vi "Write_INI.vi"(8 "error in (no error)":errorcluster, 10 "Options":T1={"Form_data_log_period"=0, "startup_threshold"=0.0, "Coeff_U"=2.55, "Offset_U"=6.5, "Coeff_I"=42.391, "Offset_I"=77.0, "Save_data_path"=path "", "ADC_frequency"=50000.0, "VISA resource name"="COM1"}, 11 "Ini_file_path":path) -> (0 "error out":errorcluster, 3 "Ini_file_path_out":path)   [LabVIEW 2012]
uses:
  Controls/options.ctl
  <vilib>/Utility/config.llb/Write Key (I32).vi
  <vilib>/Utility/config.llb/Write Key (Double).vi
  <vilib>/Utility/config.llb/Write Key (Path).vi
  <vilib>/Utility/config.llb/Write Key (String).vi
  <vilib>/Utility/config.llb/NI_LVConfig.lvlib
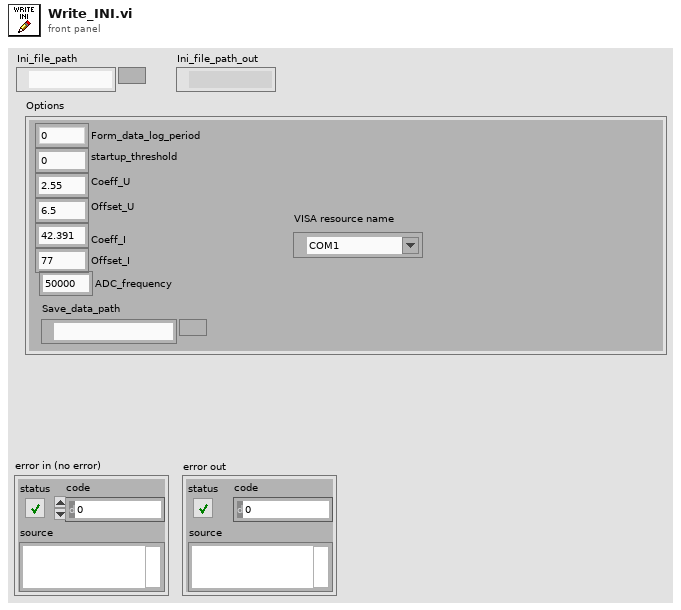
[diagram p1: front panel]
types:
  T1 = typedef "options.ctl" = cluster{"Form_data_log_period":i32, "startup_threshold":dbl, "Coeff_U":dbl, "Offset_U":dbl, "Coeff_I":dbl, "Offset_I":dbl, "Save_data_path":path, "ADC_frequency":dbl, "VISA resource name":refnum<visa-resource-name>}
  T2 = typedef "NI_LVConfig.lvlib/Config Data RefNum.ctl" = refnum<k1>
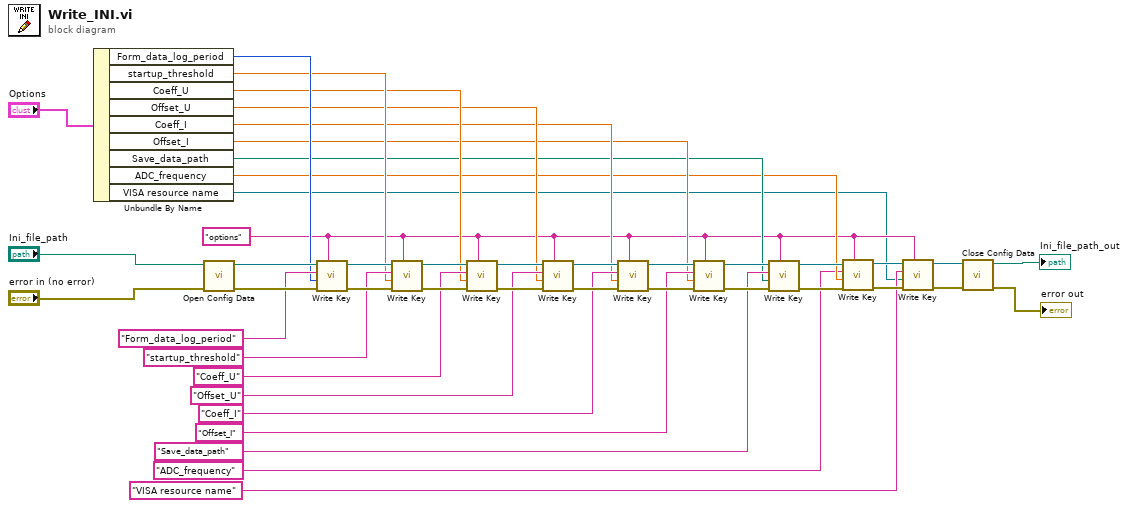
[diagram p0: block diagram]
diagram:
  w3 = "options" ("section")
  n1 = Unbundle By Name("Options") -> ("Form_data_log_period"=w36:i32, "startup_threshold"=w17:dbl, "Coeff_U"=w16:dbl, "Offset_U"=w15:dbl, "Coeff_I"=w14:dbl, "Offset_I"=w13:dbl, "Save_data_path"=w12:path, "ADC_frequency"=w9:dbl, "VISA resource name"=w1:refnum<visa-resource-name>)
  n2 = call <vilib>:"Open Config Data.vi"("error in (no error)"="error in (no error)", "configuration file path"="Ini_file_path") -> ("error out"=w42:errorcluster, "refnum"=w40:T2)  [unwired: 7 in, 1 out]
  n3 = call-poly <vilib>:"Write Key.vi"("section"=w3, "error in (no error)"=w42, "value"=w36, "key"="Form_data_log_period", "refnum"=w40) -> ("error out"=w29:errorcluster, "refnum out"=w35:T2)  [unwired: 4 in, 1 out]
  n4 = call-poly <vilib>:"Write Key.vi"("section"=w3, "error in (no error)"=w29, "value"=w17, "key"="startup_threshold", "refnum"=w35) -> ("error out"=w28:errorcluster, "refnum out"=w34:T2)  [unwired: 4 in, 1 out]
  n5 = call-poly <vilib>:"Write Key.vi"("section"=w3, "error in (no error)"=w28, "value"=w16, "key"="Coeff_U", "refnum"=w34) -> ("error out"=w27:errorcluster, "refnum out"=w33:T2)  [unwired: 4 in, 1 out]
  n6 = call-poly <vilib>:"Write Key.vi"("section"=w3, "error in (no error)"=w27, "value"=w15, "key"="Offset_U", "refnum"=w33) -> ("error out"=w26:errorcluster, "refnum out"=w32:T2)  [unwired: 4 in, 1 out]
  n7 = call-poly <vilib>:"Write Key.vi"("section"=w3, "error in (no error)"=w26, "value"=w14, "key"="Coeff_I", "refnum"=w32) -> ("error out"=w25:errorcluster, "refnum out"=w31:T2)  [unwired: 4 in, 1 out]
  n8 = call-poly <vilib>:"Write Key.vi"("section"=w3, "error in (no error)"=w25, "value"=w13, "key"="Offset_I", "refnum"=w31) -> ("error out"=w24:errorcluster, "refnum out"=w30:T2)  [unwired: 4 in, 1 out]
  n9 = call-poly <vilib>:"Write Key.vi"("section"=w3, "error in (no error)"=w24, "value"=w12, "key"="Save_data_path", "refnum"=w30) -> ("error out"=w11:errorcluster, "refnum out"=w10:T2)  [unwired: 4 in, 1 out]
  n10 = call-poly <vilib>:"Write Key.vi"("section"=w3, "error in (no error)"=w11, "value"=w9, "key"="ADC_frequency", "refnum"=w10) -> ("error out"=w7:errorcluster, "refnum out"=w5:T2)  [unwired: 4 in, 1 out]
  n11 = call-poly <vilib>:"Write Key.vi"("section"=w3, "error in (no error)"=w7, "value"=w1, "key"="VISA resource name", "refnum"=w5) -> ("error out"=w6:errorcluster, "refnum out"=w4:T2)  [unwired: 4 in, 1 out]
  n12 = call <vilib>:"Close Config Data.vi"("error in (no error)"=w6, "refnum"=w4) -> ("error out"=→"error out":errorcluster, "file path"=→"Ini_file_path_out":path)  [unwired: 8 in]
